vi "Handle Profile Resume Info.vi"(0 "Read(F)/Write(T)":bool, 7 "Current Step In":i32, 11 "Step Time Left In":dbl format="%#_13g") -> (8 "Current Step Out":i32, 15 "Step Time Left Out":dbl format="%#_13g")   [LabVIEW 2018]
uses:
  <vilib>/Utility/config.llb/Read Key (I32).vi
  <vilib>/Utility/config.llb/Read Key (Double).vi
  <vilib>/Utility/config.llb/Write Key (I32).vi
  <vilib>/Utility/config.llb/Write Key (Double).vi
  <vilib>/Utility/config.llb/NI_LVConfig.lvlib
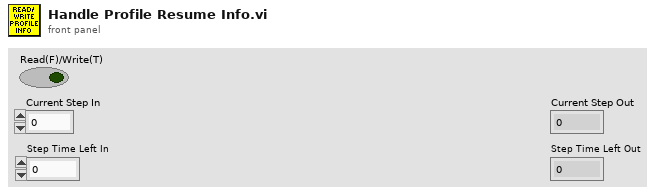
[diagram p1: front panel]
types:
  T1 = typedef "NI_LVConfig.lvlib/Config Data RefNum.ctl" = refnum<k1>
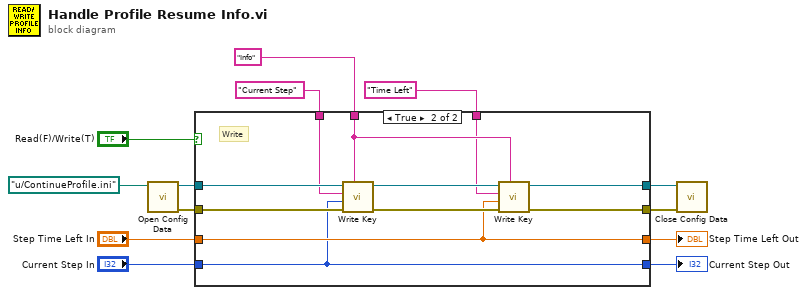
[diagram p0: block diagram]
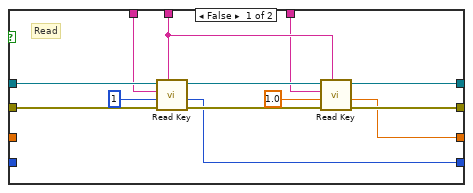
[diagram p2: hidden frame]
diagram:
  n1 = call <vilib>:"Open Config Data.vi"("configuration file path"=path "u:/ContinueProfile.ini") -> ("error out"=w9:errorcluster, "refnum"=w11:T1)  [unwired: 8 in, 1 out]
  n2 = case shown="True" "Read(F)/Write(T)" {
    tunnel: w11 -> [w26 w37]
    tunnel: [w24 w32] -> w10
    tunnel: w9 -> [w23 w36]
    tunnel: [w21 w34] -> w8
    tunnel: "Info" -> [w20 w31]
    tunnel: "Time Left" -> [w19 w30]
    tunnel: "Current Step" -> [w18 w29]
    tunnel: [w15 w27] -> w4
    tunnel: [w14 w28] -> w3
    tunnel: "Step Time Left In" -> [_ w28]
    tunnel: "Current Step In" -> [_ w27]
    frame False {
      # "Read"
      n3 = call-poly <vilib>:"Read Key.vi"("section"=w20, "error in (no error)"=w23, "default value"=1, "key"=w18, "refnum"=w26) -> ("error out"=w22:errorcluster, "value"=w15:i32, "refnum out"=w25:T1)  [unwired: 3 in, 1 out]
      n4 = call-poly <vilib>:"Read Key.vi"("section"=w20, "error in (no error)"=w22, "default value"=1.0, "key"=w19, "refnum"=w25) -> ("error out"=w21:errorcluster, "value"=w14:dbl, "refnum out"=w24:T1)  [unwired: 3 in, 1 out]
    }
    frame True {
      # "Write"
      n5 = call-poly <vilib>:"Write Key.vi"("section"=w31, "error in (no error)"=w36, "value"=w27, "key"=w29, "refnum"=w37) -> ("error out"=w35:errorcluster, "refnum out"=w33:T1)  [unwired: 4 in, 1 out]
      n6 = call-poly <vilib>:"Write Key.vi"("section"=w31, "error in (no error)"=w35, "value"=w28, "key"=w30, "refnum"=w33) -> ("error out"=w34:errorcluster, "refnum out"=w32:T1)  [unwired: 4 in, 1 out]
    }
  }
  "Current Step Out" <- w4
  "Step Time Left Out" <- w3
  n7 = call <vilib>:"Close Config Data.vi"("error in (no error)"=w8, "refnum"=w10) -> ()  [unwired: 8 in, 2 out]
